vi "StringTrimWhiteSpaces.vi"() -> ()   [LabVIEW 2019]
panel:
  out "length 2":i32
  out "length":i32
  out "trimmed string":string
  in  "String":string
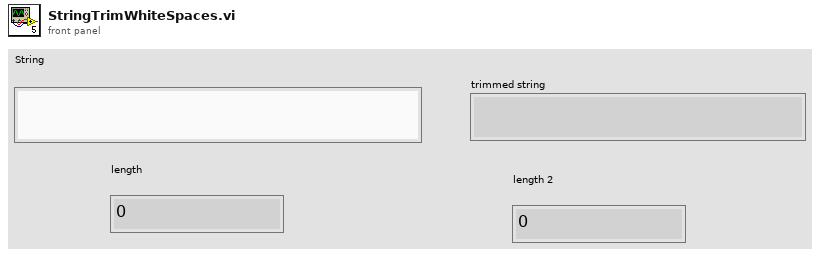
[diagram p1: front panel]
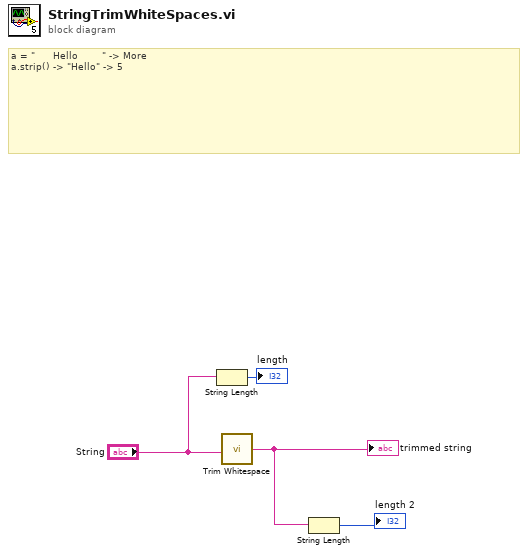
[diagram p0: block diagram]
diagram:
  # "a = \"      Hello        \" -> More\na.strip() -> \"Hello\" -> 5"
  n1 = String Length(string="String") -> (length=→"length":i32)
  n2 = call <vilib>:"Trim Whitespace.vi"("string"="String") -> ("trimmed string"=w2:string)  [unwired: 1 in]
  "trimmed string" <- w2
  n3 = String Length(string=w2) -> (length=→"length 2":i32)
